vi "Pose to Transformation Matrix.vi"(8 "error in (no error)":errorcluster, 11 "Pose":T2) -> (0 "error out":errorcluster, 3 "4x4 Transformation Matrix":T1)   [LabVIEW 2020, in "ar.lvlib"]
doc: "Convert a 3D Pose to a 4x4 Transformation Matrix. The resulting transformation matrix can be passed to \"Transformation Matrix to 3D Model View Matrix.vi\" to control the camera of a 3D Picture."
uses:
  ar.lvlib
  Pose.ctl
  rvec.ctl
  tvec.ctl
  <vilib>/Analysis/Matrix/Datatypes/RealMatrix.ctl
  Rodrigues (RVec To RMat).vi
  <vilib>/Analysis/Matrix/Numeric/Conversions/Array To Matrix.vi
  <vilib>/Analysis/Matrix/Numeric/Conversions/Array To Matrix - RA2.vi
  <vilib>/Utility/error.llb/Error Cluster From Error Code.vi
  <vilib>/Analysis/Matrix/NI_Matrix.lvlib
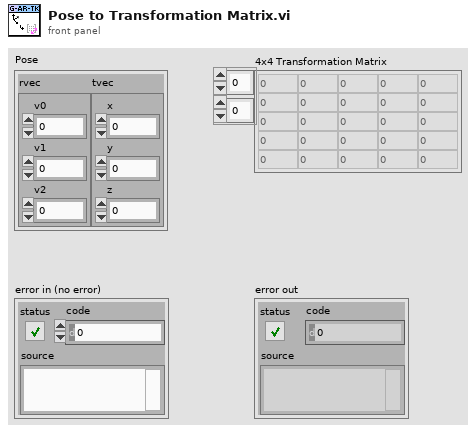
[diagram p1: front panel]
types:
  T1 = typedef "NI_Matrix.lvlib/RealMatrix.ctl" = dbl[][]
  T2 = typedef "ar.lvlib/Pose.ctl" = cluster{"rvec":T3, "tvec":T4}
  T3 = typedef "ar.lvlib/rvec.ctl" = cluster{"v0":dbl, "v1":dbl, "v2":dbl}
  T4 = typedef "ar.lvlib/tvec.ctl" = cluster{"x":dbl, "y":dbl, "z":dbl}
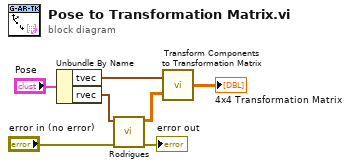
[diagram p0: block diagram]
diagram:
  n1 = Unbundle By Name("Pose") -> ("tvec"=w1:T4, "rvec"=w6:T3)
  n2 = call-poly "Rodrigues.vi"("error in (no error)"="error in (no error)", "rvec"=w6) -> ("error out"=→"error out":errorcluster, "Rotation Matrix"=w2:T1)  [unwired: 8 in]
  n3 = call "Transform Components to Transformation Matrix.vi"("Rotation Matrix in"=w2, "tvec"=w1) -> ("4x4 Transformation Matrix"=→"4x4 Transformation Matrix":T1)
